vi "fDisplay Waveform.vi"(6 "Event to display":u32, 8 "Samples per Waveform":u32=95, 9 "Location":i16(ring) items=["Purdue", "NIKHEF", "Zurich", "???"], 10 "Trigger level":i16[](array[numeric])=[4000, 4000, 4000, 4000, 4000, 4000, 4000, 4000] caption="Trigger", 11 "Waveform from DAQ":i16[](array[numeric])) -> (0 "Waveform Graph":dynamicdata(graph), 3 "Channel number displayed":i16=-1, 4 "Event displayed":i32)   [LabVIEW 2014]
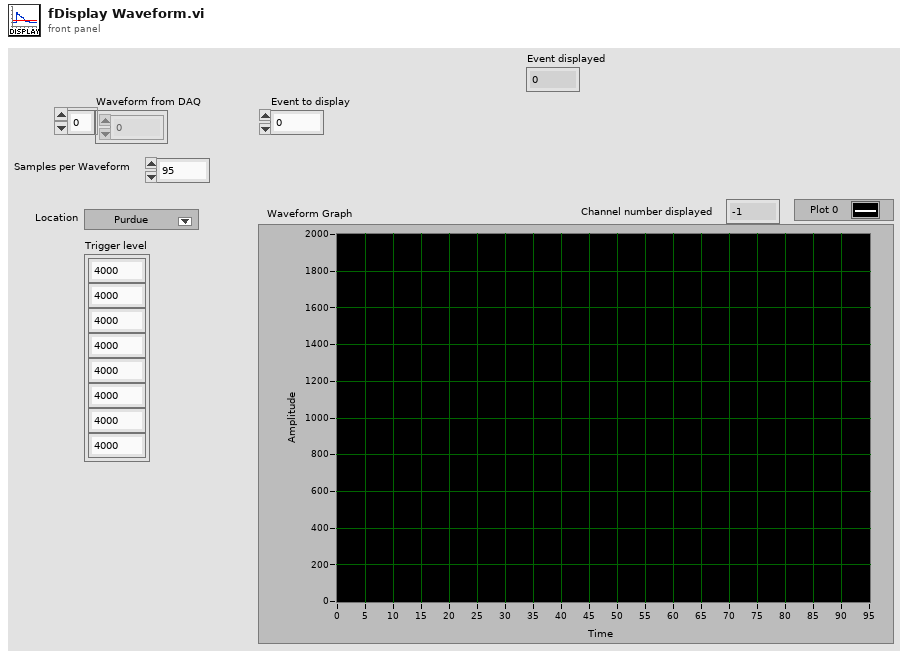
[diagram p1: front panel]
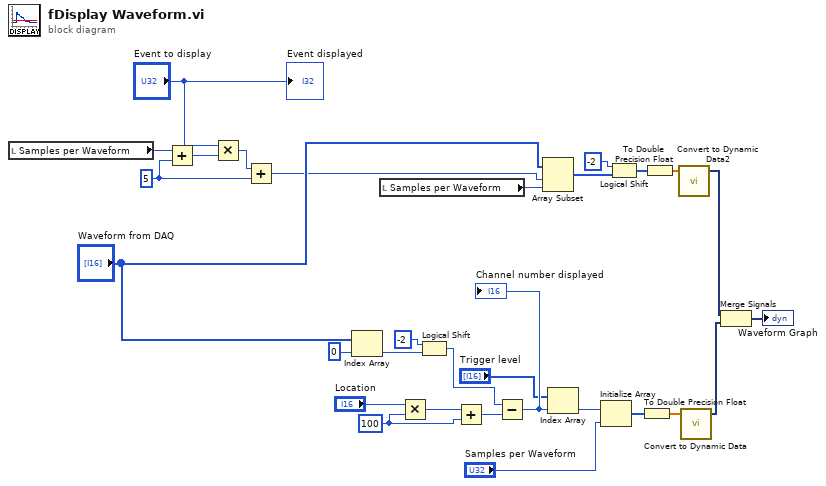
[diagram p0: block diagram]
diagram:
  w3 = 5
  w17 = i16 100
  n1 = local read "Samples per Waveform"() -> (w5:u32)
  n2 = Add(x=w5, y=w3) -> (x+y=w6:u32)
  n3 = Multiply(x="Event to display", y=w6) -> (x*y=w4:u32)
  n4 = Add(x=w4, y=w3) -> (x+y=w2:u32)
  n5 = Index Array(array="Waveform from DAQ", index=0) -> (element=w7:i16)
  n6 = local read "Samples per Waveform"() -> (w29:u32)
  n7 = Multiply(x="Location", y=w17) -> (x*y=w18:i16)
  n8 = Logical Shift(y=i16 -2, x=w7) -> (x << y=w21:i16)
  n9 = Add(x=w18, y=w17) -> (x+y=w19:i16)
  n10 = Subtract(x=w21, y=w19) -> (x-y=w11:i16)
  "Channel number displayed" <- w11
  n11 = Array Subset(array="Waveform from DAQ", index=w2, length=w29) -> (w26:i16[])
  n12 = Index Array(array="Trigger level", index=w11) -> (element=w15:i16)
  n13 = Initialize Array(w15, "Samples per Waveform") -> (w12:i16[])
  n14 = Logical Shift(y=i16 -2, x=w26) -> (x << y=w25:i16[])
  n15 = To Double Precision Float(number=w12) -> (double precision float=w16:dbl[])
  n16 = To Double Precision Float(number=w25) -> (double precision float=w28:dbl[])
  n17 = call "Convert to Dynamic Data2"("Array"=w28) -> ("Dynamic Data Type"=w23:dynamicdata)  [unwired: 3 in]
  n18 = call "Convert to Dynamic Data"("Array"=w16) -> ("Dynamic Data Type"=w13:dynamicdata)  [unwired: 3 in]
  n19 = Merge Signals(w23, w13) -> (→"Waveform Graph":dynamicdata)
  "Event displayed" <- "Event to display"
